vi "Save Test Info.vi"(1 "Parameter Table Out":string[][](array[string])) -> ()   [LabVIEW 2010]
uses:
  StateFile.llb/Actions.ctl
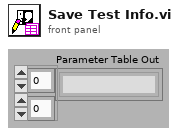
[diagram p1: front panel]
types:
  T1 = cluster{"Additional Parameter Section":string, "Blowfish Master Password":string, "Key Name":string, "Use Encryption":bool}
  T2 = typedef "Actions.ctl" = enum16{"Initialize", "Save VI State", "Load VI State", "Delete State", "Get All VI State Names", "Clear All States", "Close Global State File", "Open State File", "Create State File", "Write Data to File", "Exit"}
  T3 = typedef "Internal State Data.ctl" = cluster{"StateFile Reference":T4, "StateFile Filepath":path, "Error":errorcluster, "VI ":enum16{"By VI Name", "Calling VI"}, "VI Name":path, "State":enum16{"By State Name", "Default State"}, "State Name":string, "notifier in":refnum<notifier>, " Progress Bar":bool}
  T4 = typedef "NI_LVConfig.lvlib/Config Data RefNum.ctl" = refnum<k1>
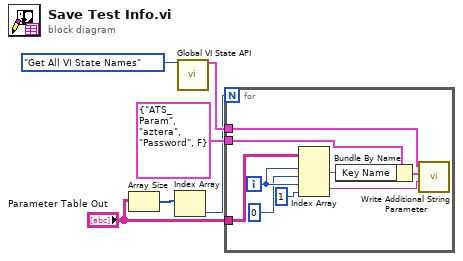
[diagram p0: block diagram]
diagram:
  n1 = Array Size(array="Parameter Table Out") -> (size(s)=w2:i32[])
  n2 = Index Array(array=w2) -> (element=w1:i32)  [unwired: 1 in]
  n3 = call "Global VI State API.vi"("Action"=Actions."Get All VI State Names") -> ("Internal State Data"=w6:T3)  [unwired: 12 in, 2 out]
  n4 = for {
    N: w1 -> [_]
    tunnel: T1 {"Additional Parameter Section"="ATS_Param", "Blowfish Master Password"="aztera", "Key Name"="Password", "Use Encryption"=FALSE} ("Additional Parameters Out") -> [w15]
    tunnel: w6 -> [w14]
    tunnel: "Parameter Table Out" -> [w12]
    i -> [w11]
    n5 = Index Array(array=w12, index (row) #1=w11, index (col) #1=0 ("disabled index (col)"), index (row) #2=w11, index (col) #2=1 ("disabled index (col)")) -> (element #1=w8:string, element #2=w7:string)
    n6 = Bundle By Name(cluster=w15, "Key Name"=w8) -> (w13:T1)
    n7 = call "Write Additional String Parameter.vi"("value"=w7, "Additional Parameters Out"=w13, "Internal State Data"=w14) -> ()  [unwired: 6 in, 3 out]
  }
